vi "Selected Plots Mouse Coordinates Constant.vi"() -> (0 "Selected Plots Mouse Coordinates Equivalent":T1={"Horizontal"=2147483647, "Vertical"=2147483647})   [LabVIEW 2021, in "Graphs.lvlib"]
uses:
  <vilib>/Utility/miscctls.llb/LVPoint32TypeDef.ctl
  Graphs.lvlib
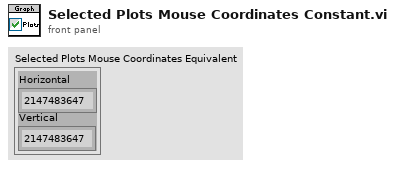
[diagram p1: front panel]
types:
  T1 = typedef "LVPoint32TypeDef.ctl" = cluster{"Horizontal":i32, "Vertical":i32}
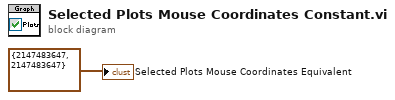
[diagram p0: block diagram]
diagram:
  "Selected Plots Mouse Coordinates Equivalent" <- T1 {"Horizontal"=2147483647, "Vertical"=2147483647} ("Mouse Click Coordinates")
